vi "plcm3ChannelSetting.vi"(0 "Handle In":i16, 1 "CH1 Measurement Type":u32(ring) items=["OFF", "1mV range (1mV/A)", "10mV range (10mV/A)", "100mV range (100mV/A)", "Voltage Input"], 2 "CH2 Measurement Type":u32(ring) items=["OFF", "1mV range (1mV/A)", "10mV range (10mV/A)", "100mV range (100mV/A)", "Voltage Input"], 3 "CH3 Measurement Type":u32(ring) items=["OFF", "1mV range (1mV/A)", "10mV range (10mV/A)", "100mV range (100mV/A)", "Voltage Input"], 11 "error in (no error)":errorcluster) -> (4 "Handle out":i16, 6 "Channel Enable Array":u8[](array[numeric]), 15 "error out":errorcluster)   [LabVIEW 2009]
uses:
  plcm3.dll
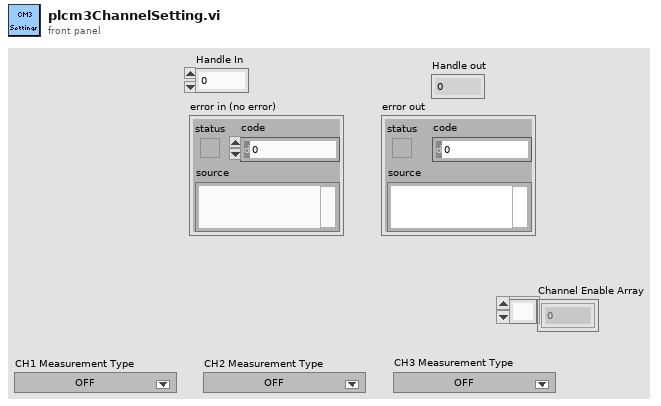
[diagram p1: front panel]
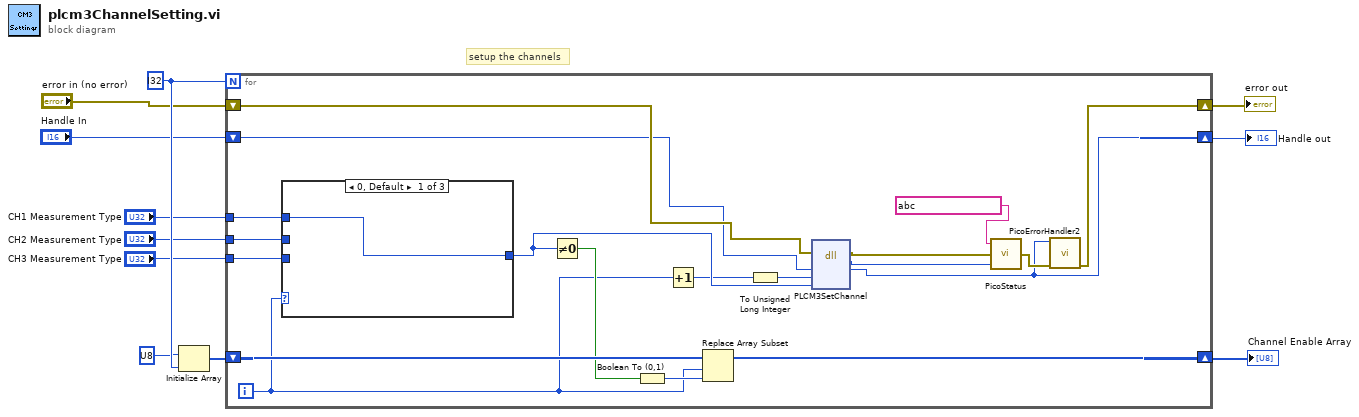
[diagram p0: block diagram]
diagram:
  w10 = i32 ?
  # "setup the channels"
  n1 = Initialize Array(u8 ? ("element"), w10) -> (w8:u8[])
  n2 = for {
    N: w10 -> [_]
    shift-right: [w30] -> w11
    shift-left: w8 -> [w29]
    shift-right: [w21] -> w7
    shift-left: "Handle In" -> [w19]
    shift-right: [w24] -> w4
    shift-left: "error in (no error)" -> [w20]
    tunnel: "CH1 Measurement Type" -> [w18]
    tunnel: "CH2 Measurement Type" -> [w16]
    tunnel: "CH3 Measurement Type" -> [w15]
    i -> [w12]
    n3 = case shown="0, Default" w12 {
      tunnel: [w31 w32 w33] -> w17
      tunnel: w18 -> [w31 _ _]
      tunnel: w16 -> [_ w32 _]
      tunnel: w15 -> [_ _ w33]
      frame #0 {
      }
      frame #1 {
      }
      frame #2 {
      }
    }
    n4 = Not Equal To 0?(x=w17) -> (x != 0?=w25:bool)
    n5 = Boolean To (0,1)(Boolean=w25) -> (0, 1=w28:i16)
    n6 = Increment(x=w12) -> (x+1=w13:i32)
    n7 = Replace Array Subset(array=w29, new element=w28, index=w12) -> (w30:u8[])
    n8 = To Unsigned Long Integer(number=w13) -> (unsigned 32bit integer=w14:u32)
    n9 = dll-call lib="PLCM3.dll" fn="PLCM3SetChannel"(error in=w20, "handle"=w19, "channel"=w14, "type"=w17) -> (error out=w23:errorcluster, "PICO_STATUS"=w22:u32, "handle"=w21:i16)  [unwired: 4 in, 1 out]
    n10 = call "PicoStatus.vi"("PICO STATUS"=w22, "error in"=w23, "source"=string ?) -> ("error out"=w27:errorcluster)
    n11 = call "PicoErrorHandler2.vi"("error in (no error)"=w27, "handle In"=w21) -> ("error out"=w24:errorcluster)  [unwired: 9 in]
  }
  "Channel Enable Array" <- w11
  "Handle out" <- w7
  "error out" <- w4
